vi "SEND READ PIN.vi"(8 "error in (no error)":errorcluster, 10 "CANAL":u8, 11 "SIMULADO in":refnum<class "SIMULADO.lvclass">) -> (0 "error out":errorcluster, 2 "read buffer":string, 3 "SIMULADO out":refnum<class "SIMULADO.lvclass">)   [LabVIEW 2019, in "SIMULADO.lvclass"]
uses:
  SIMULADO.lvclass
  MICROS.ctl
  SERIAL DEVICE/SERIAL DEVICE.lvclass
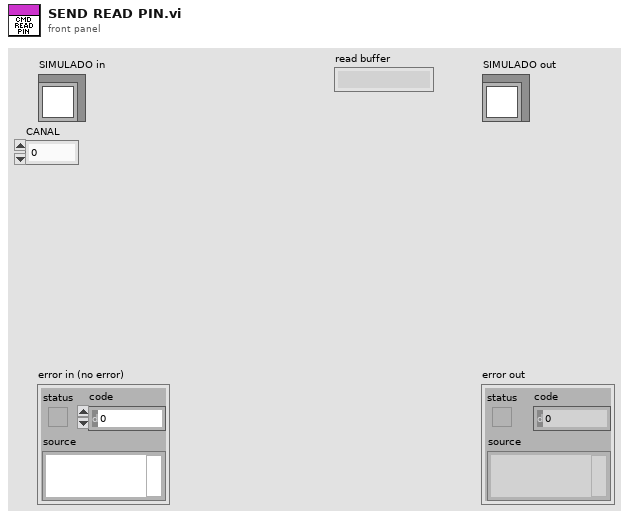
[diagram p1: front panel]
types:
  T1 = typedef "MICROS.ctl" = string
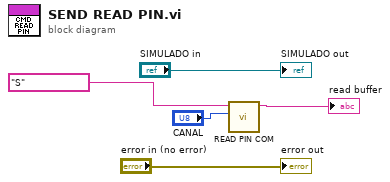
[diagram p0: block diagram]
diagram:
  n1 = call "READ PIN COM.vi"("CANAL"="CANAL", "MICROS"=T1 "S") -> ("EXPECTED RESPONSE"=→"read buffer":string)  [unwired: 7 in, 2 out]
  "error out" <- "error in (no error)"
  "SIMULADO out" <- "SIMULADO in"
